vi "ConnectRT2.vi"(8 "ErrorIn":errorcluster, 11 "Reference":T1) -> (0 "ErrorOut":errorcluster, 3 "ReferenceOut":T1)   [LabVIEW 2022 SP3]
uses:
  C:/Users/Robots/Documents/robocadSimLV/assemblies/LibraryForLabVIEW.dll
  assemblies/LibraryForLabVIEW.dll
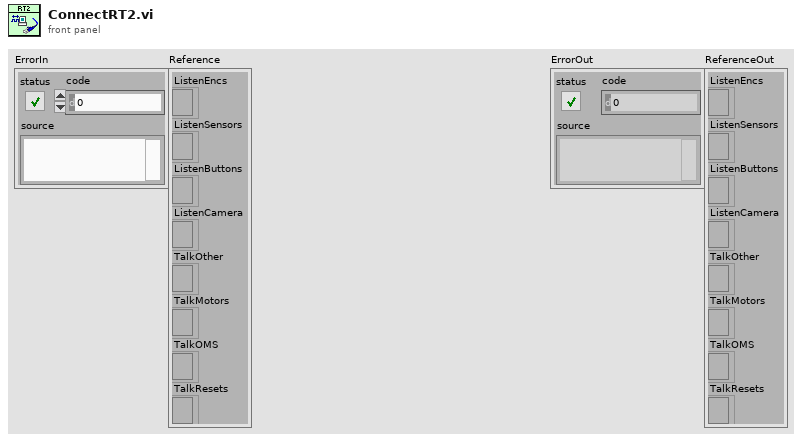
[diagram p1: front panel]
types:
  T1 = cluster{"ListenEncs":refnum<k24>, "ListenSensors":refnum<k24>, "ListenButtons":refnum<k24>, "ListenCamera":refnum<k24>, "TalkOther":refnum<k24>, "TalkMotors":refnum<k24>, "TalkOMS":refnum<k24>, "TalkResets":refnum<k24>}
  T2 = cluster{"Encs":bool, "Sensors":bool, "Buttons":bool, "Camera":bool, "Other":bool, "Motors":bool, "OMS":bool, "Resets":bool}
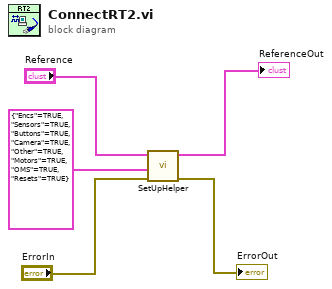
[diagram p0: block diagram]
diagram:
  n1 = call "SetUpHelper.vi"("ErrorIn"="ErrorIn", "EnableCluster"=T2 {"Encs"=TRUE, "Sensors"=TRUE, "Buttons"=TRUE, "Camera"=TRUE, "Other"=TRUE, "Motors"=TRUE, "OMS"=TRUE, "Resets"=TRUE}, "Reference"="Reference") -> ("ErrorOut"=→"ErrorOut":errorcluster, "Reference"=→"ReferenceOut":T1)  [unwired: 7 in]
